vi "Bounds.vi"(1 "XRef":refnum<vi>, 2 "State In":T2={"Input Type"=variant(dbl 0.0), "Selection"=0, "Element Names"=[], "Type Strings"=[], "Element Types"=[]}) -> (0 "Bounds":cluster{"Width":T1, "Height":T1})   [LabVIEW 2015, in "Case-Tagged-Union.xnode"]
doc: "This ability VI is used to tell LabVIEW your current bounds. If you want to update your bounds, you must inform LabVIEW through the UpdateImageAndBounds reply of another ability VI. If you change your bounds, you will also probably want to update your image.\n\nDefault behavior: None.\n\nThis ability does not provide UI and OS messages are not handled."
uses:
  Case-Tagged-Union.xnode
  State.ctl
  <vilib>/XNodeSupport/XNodeInt.ctl
  <vilib>/XNodeSupport/NI_XNodeSupport.lvlib
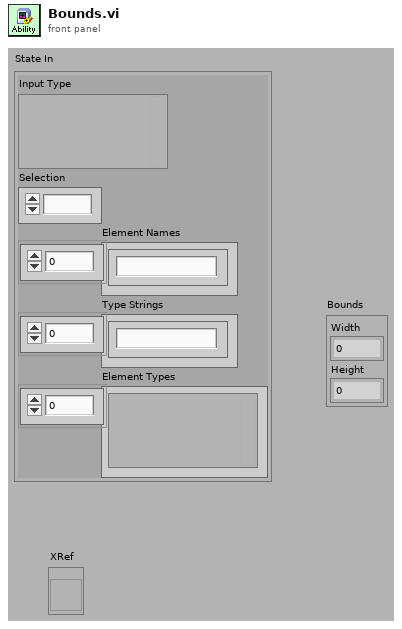
[diagram p1: front panel]
types:
  T1 = typedef "NI_XNodeSupport.lvlib/XNodeInt.ctl" = i32
  T2 = typedef "Case-Tagged-Union.xnode/State.ctl" = cluster{"Input Type":variant, "Selection":i32, "Element Names":string[], "Type Strings":string[], "Element Types":variant[]}
  T3 = cluster{"left":i16, "top":i16, "right":i16, "bottom":i16}
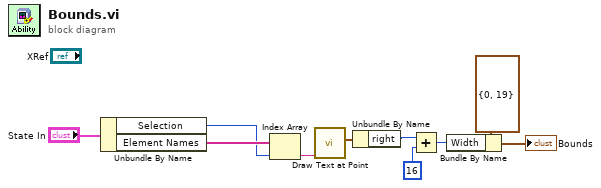
[diagram p0: block diagram]
diagram:
  n1 = Unbundle By Name("State In") -> ("Selection"=w2:i32, "Element Names"=w7:string[])
  n2 = Index Array(array=w7, index=w2) -> (element=w6:string)
  n3 = call <vilib>:"Draw Text at Point.vi"("text"=w6) -> ("text rect"=w5:T3)  [unwired: 9 in, 1 out]
  n4 = Unbundle By Name(w5) -> ("right"=w4:i16)
  n5 = Add(x=w4, y=i16 16) -> (x+y=w3:i16)
  n6 = Bundle By Name(cluster=cluster{"Width":T1, "Height":T1} {"Width"=0, "Height"=19} ("Bounds"), "Width"=w3) -> (→"Bounds":cluster{"Width":T1, "Height":T1})
